vi "System Reporting.vi"(8 "Error In":errorcluster, 10 "String":string, 11 "Byte Stream File in":refnum<file>) -> (0 "Error Out":errorcluster, 3 "Byte Stream File out":refnum<file>)   [LabVIEW 2020]
doc: "Author: Scott Hannahs <sth@magnet.fsu.edu>\nCopyright 2018 Florida State University, All rights reserved."
uses:
  <vilib>/Utility/error.llb/DialogType.ctl
  RT Host Globals.vi
  <vilib>/regexp/Match Regular Expression.xnode
  <vilib>/NI_Real-Time Target Support.lvlib
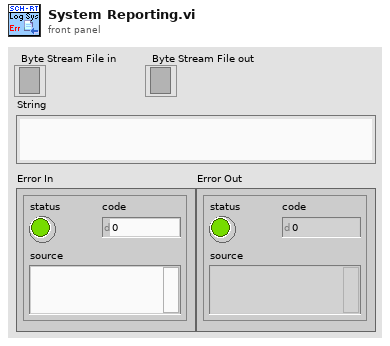
[diagram p1: front panel]
types:
  T1 = enum16{"open", "replace", "create", "open or create", "replace or create", "replace or create with confirmation"}
  T2 = typedef "NI_Real-Time Target Support.lvlib/RT CPU Load.ctl" = cluster{"Total (%)":dbl, "Time Critical (%)":dbl, "Timed Structures (%)":dbl, "High (%)":dbl, "Above Normal (%)":dbl, "Normal (%)":dbl, "Background (%)":dbl, "Idle (%)":dbl, "ISR (%)":dbl}
  T3 = typedef "DialogType.ctl" = u16
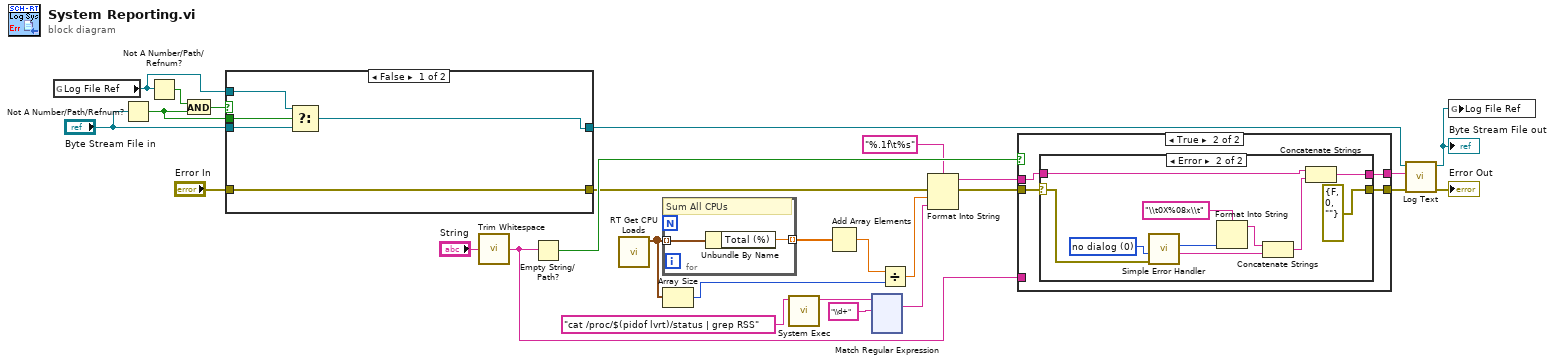
[diagram p0: block diagram]
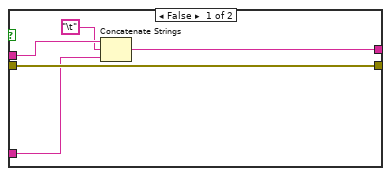
[diagram p2: hidden frame]
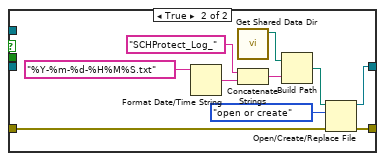
[diagram p4: hidden frame]
diagram:
  n1 = global read "RT Host Globals.vi" "Log File Ref"() -> (w17:refnum<file>)
  n2 = Not A Number/Path/Refnum?(number/path/refnum="Byte Stream File in") -> (NaN/Path/Refnum?=w16:bool)
  n3 = Not A Number/Path/Refnum?(number/path/refnum=w17) -> (NaN/Path/Refnum?=w19:bool)
  n4 = And(x=w19, y=w16) -> (x .and. y?=w20:bool)
  n5 = case shown="False" w20 {
    tunnel: [w31 w42] -> w18
    tunnel: "Byte Stream File in" -> [w30 _]
    tunnel: [w32 w34] -> w2
    tunnel: "Error In" -> [w32 w33]
    tunnel: w17 -> [w29 _]
    tunnel: w16 -> [w28 _]
    frame False {
      n6 = Select(t=w29, s=w28, f=w30) -> (s? t:f=w31:refnum<file>)
    }
    frame True {
      n7 = Format Date/Time String(time format string (%c)="%Y-%m-%d-%H%M%S.txt") -> (date/time string=w35:string)  [unwired: 2 in]
      n8 = call "Get Shared Data Dir.vi"() -> ("Data Directory Path"=w41:path)  [unwired: 2 in, 1 out]
      n9 = Concatenate Strings("SCHProtect_Log_" ("name or relative path"), w35) -> (w36:string)
      n10 = Build Path(base path=w41, name or relative path=w36) -> (appended path=w39:path)
      n11 = Open/Create/Replace File(file path (use dialog)=w39, error in=w33, operation (0:open)=T1."open or create") -> (refnum out=w42:refnum<file>, error out=w34:errorcluster)  [unwired: 3 in, 1 out]
    }
  }
  n12 = call <vilib>:"Trim Whitespace.vi"("string"="String") -> ("trimmed string"=w15:string)  [unwired: 1 in]
  n13 = Empty String/Path?(string/path=w15) -> (empty?=w24:bool)
  n14 = call <vilib>:"RT Get CPU Loads.vi"() -> ("CPU loads"=w10:T2[])  [unwired: 10 in, 1 out]
  n15 = for {
    tunnel: w10 -> [w44] mode=indexing
    tunnel: [w43] -> w9 mode=indexing
    # "Sum All CPUs"
    n16 = Unbundle By Name(w44) -> ("Total (%)"=w43:dbl)
  }
  n17 = Array Size(array=w10) -> (size(s)=w7:i32)
  n18 = call <vilib>:"System Exec.vi"("command line"="cat /proc/$(pidof lvrt)/status | grep RSS") -> ("standard output"=w5:string)  [unwired: 7 in, 3 out]
  n19 = Add Array Elements(numeric array=w9) -> (sum=w8:dbl)
  n20 = xnode "Match Regular Expression"("input string"=w5, "regular expression"="\\d+") -> ("whole match"=w4:string)  [unwired: 4 in, 4 out]
  n21 = Divide(x=w8, y=w7) -> (x/y=w6:dbl)
  n22 = Format Into String(format string="%.1f\t%s", error in=w2, w6, w4) -> (resulting string=w1:string, error out=w3:errorcluster)  [unwired: 1 in]
  n23 = case shown="True" w24 {
    tunnel: w3 -> [w49 w51]
    tunnel: [w48 w53] -> w23
    tunnel: [w49 w52] -> w22
    tunnel: w15 -> [w46 _]
    tunnel: w1 -> [w47 w50]
    frame False {
      n24 = Concatenate Strings(w47, "\t", w46) -> (w48:string)
    }
    frame True {
      n25 = case shown="Error" w51 {
        selector: w51 -> [w55 w63]
        tunnel: [w54 w57] -> w53
        tunnel: [w55 errorcluster {"status"=FALSE, "code"=0, "source"=""} ("error IO")] -> w52
        tunnel: w50 -> [w54 w56]
        frame No Error {
        }
        frame Error {
          w65 = T3 0 items=["no dialog", "OK message", "continue or stop message", "OK message + warnings", "continue/stop + warnings"] ("type of dialog (OK msg:1)")
          n26 = call <vilib>:"Simple Error Handler.vi"("type of dialog (OK msg:1)"=w65, "error in (no error)"=w63) -> ("code out"=w59:i32, "source out"=w62:string)  [unwired: 3 in, 3 out]
          n27 = Format Into String(format string="\\t0X%08x\\t", w59) -> (resulting string=w60:string)  [unwired: 2 in, 1 out]
          n28 = Concatenate Strings(w60, w62) -> (w61:string)
          n29 = Concatenate Strings(w56, w61) -> (w57:string)
        }
      }
    }
  }
  n30 = call "Log Text.vi"("Error In"=w22, "text"=w23, "Log File Ref In"=w18) -> ("Error Out"=→"Error Out":errorcluster, "Log File Ref Out"=w14:refnum<file>)  [unwired: 7 in]
  "Byte Stream File out" <- w14
  n31 = global write "RT Host Globals.vi" "Log File Ref"(w14) -> ()
